vi "加标模块单控对话框.vi"(10 "数组":refnum<vi>[](array[refnum]), 11 "标题":string="加标模块") -> ()   [LabVIEW 2016, in "质控单元.lvlib"]
panel:
  in  "慢速到液位":bool
  in  "排液":bool
  in  "退出":bool
  in  "柱塞泵":bool
  in  "排液":bool
  in  "搅拌":bool
  in  "进样调速":bool
  in  "进样":bool
  in  "停止":bool
  in  "加标启动":bool
  # "手动控制"
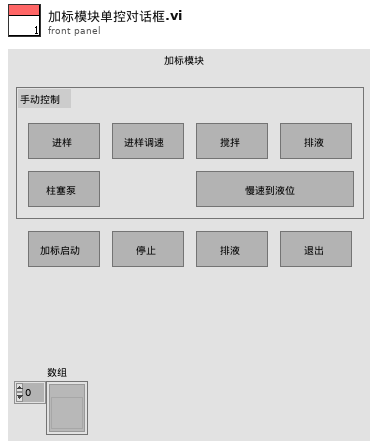
[diagram p1: front panel]
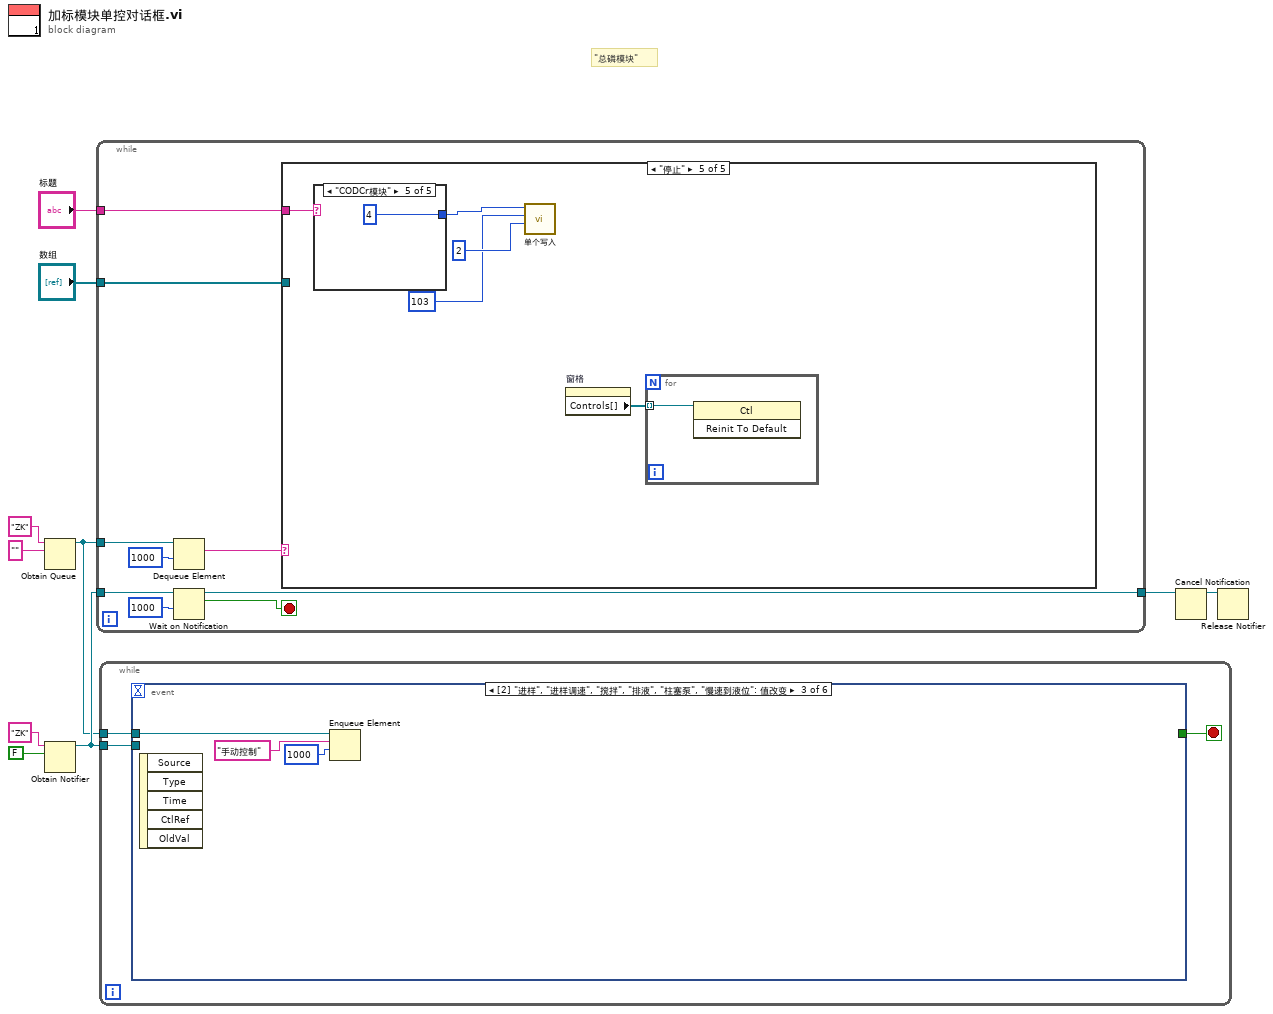
[diagram p0: block diagram]
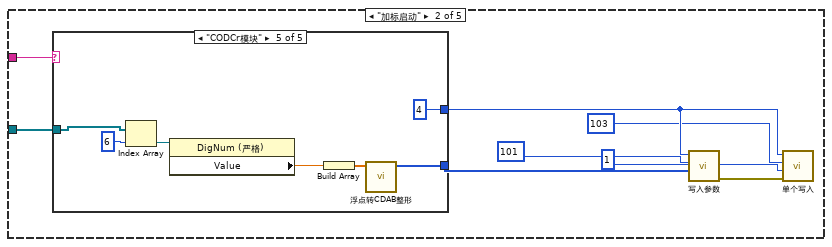
[diagram p3: hidden frame]
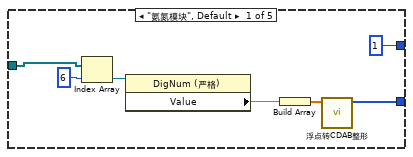
[diagram p4: hidden frame]
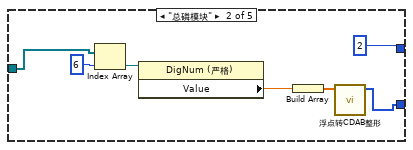
[diagram p5: hidden frame]
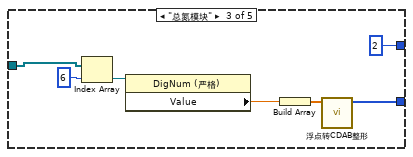
[diagram p6: hidden frame]
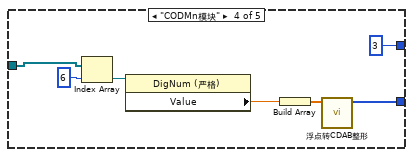
[diagram p7: hidden frame]
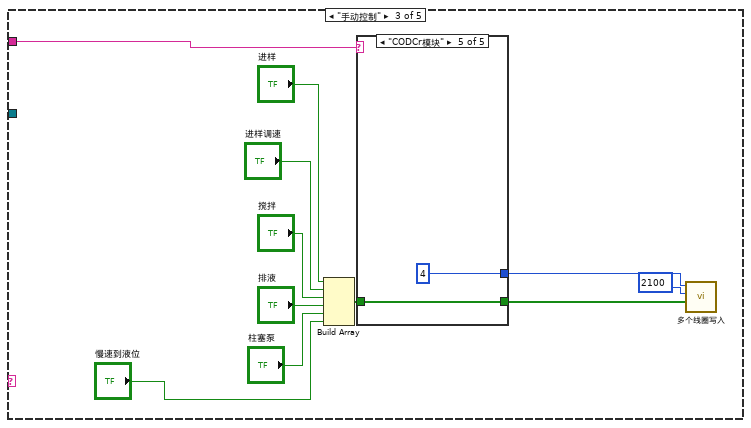
[diagram p8: hidden frame]
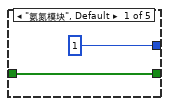
[diagram p9: hidden frame]
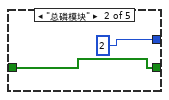
[diagram p10: hidden frame]
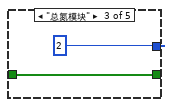
[diagram p11: hidden frame]
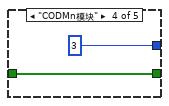
[diagram p12: hidden frame]
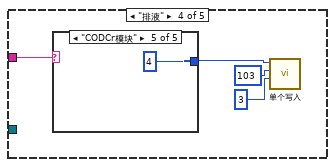
[diagram p13: hidden frame]
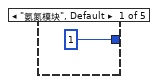
[diagram p14: hidden frame]
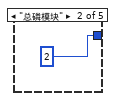
[diagram p15: hidden frame]
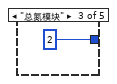
[diagram p16: hidden frame]
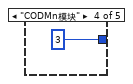
[diagram p17: hidden frame]
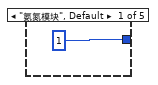
[diagram p18: hidden frame]
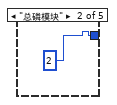
[diagram p19: hidden frame]
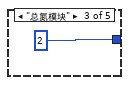
[diagram p20: hidden frame]
diagram:
  # "\"总磷模块\""
  n1 = Obtain Queue(name (unnamed)="ZK" ("名称（未命名）"), element data type="" ("名称（未命名）")) -> (queue out=w3:refnum<queue>)  [unwired: 3 in, 2 out]
  n2 = Obtain Notifier(name (unnamed)="ZK" ("名称（未命名）"), notification data type=FALSE) -> (notifier out=w8:refnum<notifier>)  [unwired: 2 in, 2 out]
  n3 = while {
    tunnel: w8 -> [w19]
    tunnel: [w17] -> w7
    tunnel: w3 -> [w16]
    tunnel: "数组" -> [w11]
    tunnel: "标题" -> [w12]
    stop <- w18 stop-if-true
    n4 = Dequeue Element(queue=w16, timeout in ms (-1)=1000 ("超时毫秒(-1)")) -> (element=w15:string)  [unwired: 1 in, 3 out]
    n5 = Wait on Notification(notifier=w19, timeout in ms (-1)=1000 ("超时毫秒(-1)")) -> (notifier out=w17:refnum<notifier>, notification=w18:bool)  [unwired: 2 in, 2 out]
    n6 = case shown="\"停止\"" w15 {
      tunnel: w12 -> [_ w21 w63 w84 w94]
      tunnel: w11 -> [_ w20 _ _ _]
      frame Default {
      }
      frame "加标启动" {
        n7 = case shown="\"CODCr模块\"" w21 {
          tunnel: w20 -> [w30 w41 w44 w51 w58]
          tunnel: [w29 w40 w43 w50 w57] -> w23
          tunnel: [u8 1 ("Slave ID") u8 2 ("Slave ID") u8 2 ("Slave ID") u8 3 ("Slave ID") u8 4 ("Slave ID")] -> w27
          frame "氨氮模块", Default {
            n8 = Index Array(array=w30, index=6 ("索引")) -> (element=w34:refnum<vi>)
            n9 = property class="DigNum (严格)"(reference=w34) -> ("Value"=w33:dbl)  [unwired: 1 in, 2 out]
            n10 = Build Array(w33) -> (w32:dbl[])
            n11 = call "浮点转CDAB整形.vi"("浮点数"=w32) -> ("CDAB整形输出"=w29:u16[])  [unwired: 10 in]
          }
          frame "总磷模块" {
            n12 = Index Array(array=w41, index=6 ("索引")) -> (element=w38:refnum<vi>)
            n13 = property class="DigNum (严格)"(reference=w38) -> ("Value"=w37:dbl)  [unwired: 1 in, 2 out]
            n14 = Build Array(w37) -> (w36:dbl[])
            n15 = call "浮点转CDAB整形.vi"("浮点数"=w36) -> ("CDAB整形输出"=w40:u16[])  [unwired: 10 in]
          }
          frame "总氮模块" {
            n16 = Index Array(array=w44, index=6 ("索引")) -> (element=w48:refnum<vi>)
            n17 = property class="DigNum (严格)"(reference=w48) -> ("Value"=w47:dbl)  [unwired: 1 in, 2 out]
            n18 = Build Array(w47) -> (w46:dbl[])
            n19 = call "浮点转CDAB整形.vi"("浮点数"=w46) -> ("CDAB整形输出"=w43:u16[])  [unwired: 10 in]
          }
          frame "CODMn模块" {
            n20 = Index Array(array=w51, index=6 ("索引")) -> (element=w55:refnum<vi>)
            n21 = property class="DigNum (严格)"(reference=w55) -> ("Value"=w54:dbl)  [unwired: 1 in, 2 out]
            n22 = Build Array(w54) -> (w53:dbl[])
            n23 = call "浮点转CDAB整形.vi"("浮点数"=w53) -> ("CDAB整形输出"=w50:u16[])  [unwired: 10 in]
          }
          frame "CODCr模块" {
            n24 = Index Array(array=w58, index=6 ("索引")) -> (element=w62:refnum<vi>)
            n25 = property class="DigNum (严格)"(reference=w62) -> ("Value"=w61:dbl)  [unwired: 1 in, 2 out]
            n26 = Build Array(w61) -> (w60:dbl[])
            n27 = call "浮点转CDAB整形.vi"("浮点数"=w60) -> ("CDAB整形输出"=w57:u16[])  [unwired: 10 in]
          }
        }
        n28 = call "写入参数.vi"("values"=w23, "starting address"=u16 101, "Slave ID"=w27) -> ("error out"=w22:errorcluster)  [unwired: 8 in]
        n29 = call "单个写入.vi"("Error in"=w22, "value"=u16 1, "address"=u16 103, "Slave ID"=w27) -> ()  [unwired: 7 in, 1 out]
      }
      frame "手动控制" {
        n30 = Build Array("进样", "进样调速", "搅拌", "排液", "柱塞泵", "慢速到液位") -> (w69:bool[])
        n31 = case shown="\"CODCr模块\"" w63 {
          tunnel: w69 -> [w75 w77 w78 w81 w83]
          tunnel: [w75 w77 w78 w81 w83] -> w70
          tunnel: [u8 1 ("Slave ID") u8 2 ("Slave ID") u8 2 ("Slave ID") u8 3 ("Slave ID") u8 4 ("Slave ID")] -> w72
          frame "氨氮模块", Default {
          }
          frame "总磷模块" {
          }
          frame "总氮模块" {
          }
          frame "CODMn模块" {
          }
          frame "CODCr模块" {
          }
        }
        n32 = call "多个线圈写入.vi"("values"=w70, "starting address"=u16 2100, "Slave ID"=w72) -> ()  [unwired: 8 in, 1 out]
      }
      frame "排液" {
        n33 = case shown="\"CODCr模块\"" w84 {
          tunnel: [u8 1 ("Slave ID") u8 2 ("Slave ID") u8 2 ("Slave ID") u8 3 ("Slave ID") u8 4 ("Slave ID")] -> w85
          frame "氨氮模块", Default {
          }
          frame "总磷模块" {
          }
          frame "总氮模块" {
          }
          frame "CODMn模块" {
          }
          frame "CODCr模块" {
          }
        }
        n34 = call "单个写入.vi"("value"=u16 3, "address"=u16 103, "Slave ID"=w85) -> ()  [unwired: 8 in, 1 out]
      }
      frame "停止" {
        n35 = case shown="\"CODCr模块\"" w94 {
          tunnel: [u8 1 ("Slave ID") u8 2 ("Slave ID") u8 2 ("Slave ID") u8 3 ("Slave ID") u8 4 ("Slave ID")] -> w95
          frame "氨氮模块", Default {
          }
          frame "总磷模块" {
          }
          frame "总氮模块" {
          }
          frame "CODMn模块" {
          }
          frame "CODCr模块" {
          }
        }
        n36 = call "单个写入.vi"("value"=u16 2, "address"=u16 103, "Slave ID"=w95) -> ()  [unwired: 8 in, 1 out]
        n37 = property on="窗格" class="Pane"() -> ("Controls[]"=w93:refnum<vi>[])  [unwired: 2 in, 2 out]
        n38 = for {
          tunnel: w93 -> [w98] mode=indexing
          n39 = invoke class="Ctl" method="Reinit To Default"(reference=w98) -> ()  [unwired: 2 in, 3 out]
        }
      }
    }
  }
  n40 = while {
    tunnel: w8 -> [w105]
    tunnel: w3 -> [w104]
    stop <- w106 stop-if-true
    n41 = event shown="[2] \"进样\", \"进样调速\", \"搅拌\", \"排液\", \"柱塞泵\", \"慢速到液位\": 值改变" {
      selector: _ -> [_ _ _ _ _ _]
      dyn-events: _ -> [_ _ _ _ _ _]
      timeout: _ -> [_ _ _ _ _ _]
      tunnel: [_ _ _ _ _ TRUE] -> w106
      tunnel: w105 -> [_ _ _ _ _ w122]
      tunnel: w104 -> [_ w109 w110 w113 w118 w121]
      event Timeout {
        n42 = event-data() -> ()  [unwired: 1 in, 3 out]
      }
      event "加标启动": Value Change {
        n43 = event-data() -> ()  [unwired: 1 in, 4 out]
        n44 = Enqueue Element(queue=w109, element="加标启动" ("元素"), timeout in ms (-1)=1000 ("超时毫秒(-1)")) -> ()  [unwired: 1 in, 3 out]
      }
      event "进样", "进样调速", "搅拌", "排液", "柱塞泵", "慢速到液位": Value Change {
        n45 = event-data() -> ()  [unwired: 1 in, 5 out]
        n46 = Enqueue Element(queue=w110, element="手动控制" ("元素"), timeout in ms (-1)=1000 ("超时毫秒(-1)")) -> ()  [unwired: 1 in, 3 out]
      }
      event "排液": Value Change {
        n47 = event-data() -> ()  [unwired: 1 in, 6 out]
        n48 = Enqueue Element(queue=w113, element="排液" ("元素"), timeout in ms (-1)=1000 ("超时毫秒(-1)")) -> ()  [unwired: 1 in, 3 out]
      }
      event "停止": Value Change {
        n49 = event-data() -> ()  [unwired: 1 in, 5 out]
        n50 = Flush Queue(queue=w118) -> (queue out=w117:refnum<queue>)  [unwired: 1 in, 2 out]
        n51 = Enqueue Element(queue=w117, element="停止" ("元素"), timeout in ms (-1)=1000 ("超时毫秒(-1)")) -> ()  [unwired: 1 in, 3 out]
      }
      event "退出": Value Change; Panel Close {
        n52 = event-data() -> ()  [unwired: 1 in, 3 out]
        n53 = Send Notification(notification=TRUE ("通知"), notifier=w122) -> ()  [unwired: 1 in, 2 out]
        n54 = Flush Queue(queue=w121) -> (queue out=w120:refnum<queue>)  [unwired: 1 in, 2 out]
        n55 = Two Button Dialog(message="请确认是否退出，退出仪器将停止运行" ("消息"), 1:"N" ("F按钮名称（“取消”）"), 2:"Y" ("T按钮名称（“确定”）")) -> (T button?=w124:bool)
        n56 = case shown="真" w124 {
          tunnel: w120 -> [_ w129]
          frame False {
          }
          frame True {
            n57 = property on="窗格" class="Pane"() -> ("Controls[]"=w132:refnum<vi>[])  [unwired: 2 in, 2 out]
            n58 = Enqueue Element(queue=w129, element="停止" ("元素"), timeout in ms (-1)=1000 ("超时毫秒(-1)")) -> ()  [unwired: 1 in, 3 out]
            n59 = for {
              tunnel: w132 -> [w133] mode=indexing
              n60 = invoke class="Ctl" method="Reinit To Default"(reference=w133) -> ()  [unwired: 2 in, 3 out]
            }
          }
        }
      }
    }
  }
  n61 = Cancel Notification(0:w7) -> (8:w6:refnum<notifier>)  [unwired: 1 in, 2 out]
  n62 = Release Notifier(notifier=w6) -> ()  [unwired: 2 in, 3 out]
